vi "Create Message - Trigger Only.vi"(7 "optional settings":T2={"Protection"=enum."None", "Enable Periodic Default"=FALSE, "Trigger Channel refnum"=18446744073709551615} {"Trigger Channel refnum" format="%x"}, 8 "error in (no error)":errorcluster, 10 "message name":string, 11 "message group refnum in":T1=18446744073709551615 format="%.0x") -> (0 "error out":errorcluster, 2 "message refnum out":T1 format="%.0x", 3 "message group refnum out":T1 format="%.0x")   [LabVIEW 2020, in "Instrument Addon Scripting API.lvlib"]
doc: "Creates a new message section that sets the Generation Type as Trigger Only. \n\nTrigger Only is best used for single event messages, such as setting the instrument configuration at the beginning of a test."
uses:
  Instrument Addon Scripting API.lvlib
  TypeDefs/Message Settings.ctl
  TypeDefs/Protection Types.ctl
  <vilib>/NI VeriStand/Custom Device API/Custom Device Item Ref.ctl
  <vilib>/NI VeriStand/Custom Device API/Custom Device Channel.ctl
  <vilib>/NI VeriStand/Custom Device API/Custom Device Channel Type.ctl
  Addon/Addon Shared/Types/Message Generation Type.ctl
  <vilib>/NI VeriStand/Custom Device API/Custom Device API.lvlib
  Addon/Addon Shared/Instrument Addon Shared.lvlib
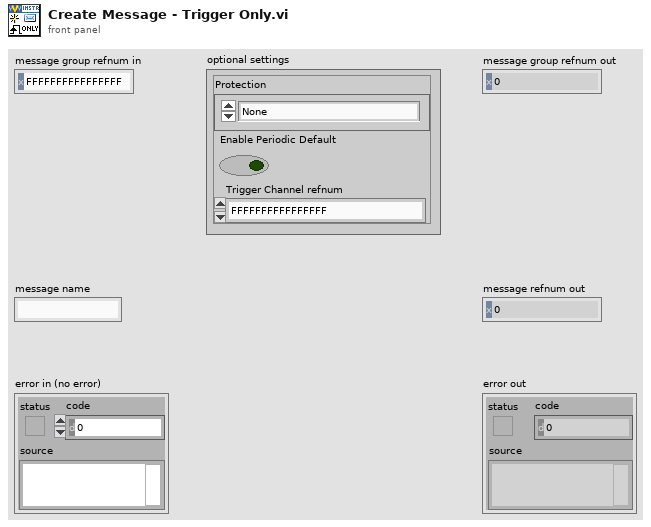
[diagram p1: front panel]
types:
  T1 = typedef "Custom Device API.lvlib/Custom Device Item Ref.ctl" = u64
  T2 = typedef "Instrument Addon Scripting API.lvlib/Message Settings.ctl" = cluster{"Protection":T3, "Enable Periodic Default":bool, "Trigger Channel refnum":u64}
  T3 = typedef "Instrument Addon Scripting API.lvlib/Protection Types.ctl" = enum16{"None", "CRC-32", "Checksum U16", "Checksum U32", "Checksum U8"}
  T4 = typedef "Instrument Addon Shared.lvlib/Message Generation Type.ctl" = enum16{"Trigger Only", "Periodic & Trigger", "Value Change & Trigger"}
  T5 = typedef "Custom Device API.lvlib/Custom Device Channel.ctl" = cluster{"Type":T6, "Units":string, "Default Value":dbl, "Faultable":bool, "Scalable":bool}
  T6 = typedef "Custom Device API.lvlib/Custom Device Channel Type.ctl" = enum16{"Input", "Output"}
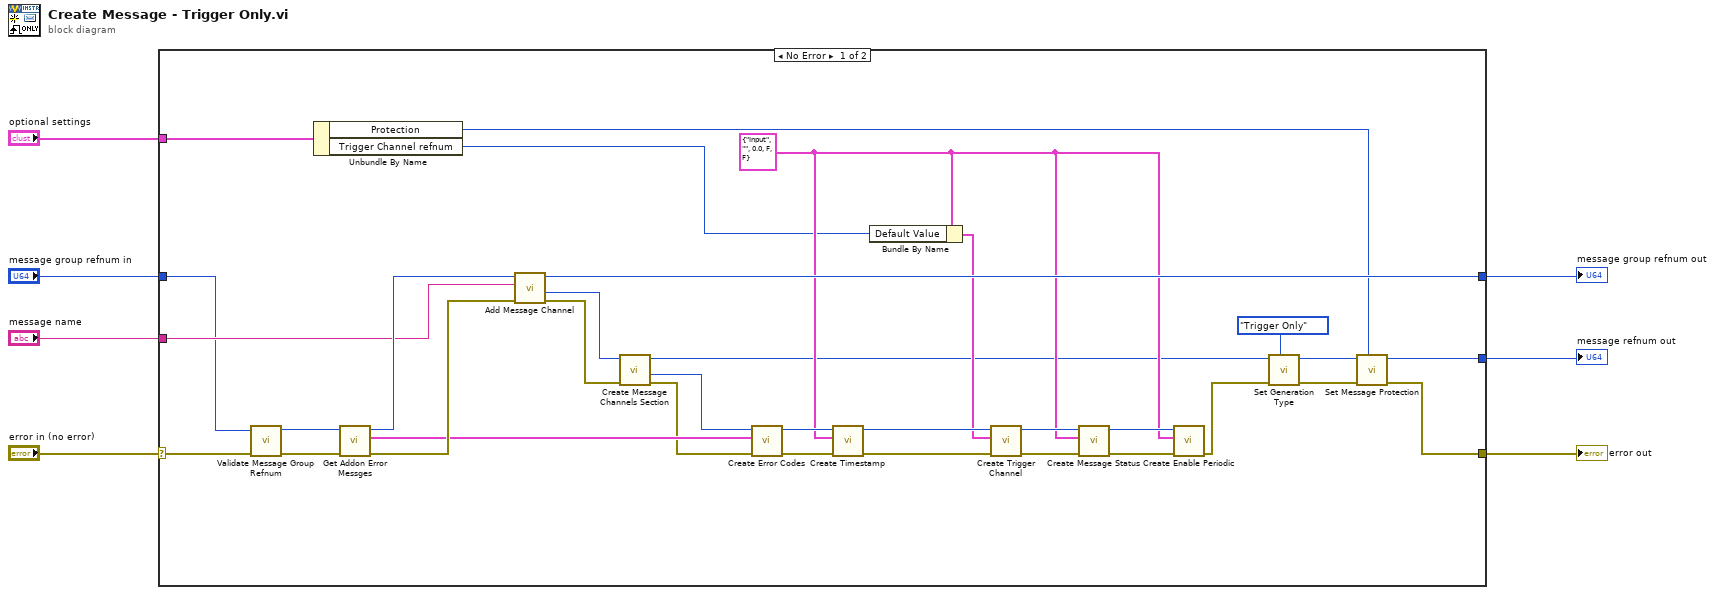
[diagram p0: block diagram]
diagram:
  n1 = case shown="No Error" "error in (no error)" {
    selector: "error in (no error)" -> [w10 w42]
    tunnel: "message group refnum in" -> [w9 w41]
    tunnel: "optional settings" -> [w36 _]
    tunnel: [w32 w41] -> w3
    tunnel: "message name" -> [w29 _]
    tunnel: [w24 _] -> w2
    tunnel: [w23 w42] -> w7
    frame No Error {
      w16 = T5 {"Type"=enum."Input", "Units"="", "Default Value"=0.0, "Faultable"=FALSE, "Scalable"=FALSE} ("Channel")
      n2 = call "Validate Message Group Refnum.vi"("error in (no error)"=w10, "message group refnum in"=w9) -> ("error out"=w11:errorcluster, "message group refnum out"=w8:T1)  [unwired: 8 in]
      n3 = Unbundle By Name(w36) -> ("Protection"=w25:T3, "Trigger Channel refnum"=w14:u64)
      n4 = call "Get Addon Error Messges.vi"("error in (no error)"=w11, "Message Group in"=w8) -> ("error out"=w37:errorcluster, "Error Messages out"=w34:cluster{"Code":i32, "String":string}[], "Message Group out"=w33:u64)  [unwired: 7 in]
      n5 = call "Add Message Channel.vi"("error in (no error)"=w37, "Message Name"=w29, "Message Group in"=w33) -> ("error out"=w40:errorcluster, "Message out"=w35:T1, "Message Group out"=w32:T1)  [unwired: 6 in]
      n6 = call "Create Message Channels Section.vi"("error in (no error)"=w40, "Message in"=w35) -> ("error out"=w31:errorcluster, "Message Channels Section out"=w30:T1, "Message out"=w12:T1)  [unwired: 7 in]
      n7 = call "Create Error Codes.vi"("error in (no error)"=w31, "Error Codes"=w34, "Message Channels Section in"=w30) -> ("error out"=w22:errorcluster, "Message Channels Section out"=w21:T1)  [unwired: 7 in]
      n8 = call "Create Timestamp.vi"("error in (no error)"=w22, "Channel Paramters"=w16, "Message Channels Section in"=w21) -> ("error out"=w20:errorcluster, "Message Channels Section out"=w19:T1)  [unwired: 6 in, 1 out]
      n9 = Bundle By Name(cluster=w16, "Default Value"=w14) -> (w15:T5)
      n10 = call "Create Trigger Channel.vi"("error in (no error)"=w20, "Channel Parameters"=w15, "Message Channels Section in"=w19) -> ("error out"=w18:errorcluster, "Message Channels Section out"=w17:T1)  [unwired: 6 in, 1 out]
      n11 = call "Create Message Status.vi"("error in (no error)"=w18, "Channel Paramters"=w16, "Message Channels Section in"=w17) -> ("error out"=w39:errorcluster, "Message Channels Section out"=w38:T1)  [unwired: 7 in]
      n12 = call "Create Enable Periodic.vi"("error in (no error)"=w39, "Channel Parameters"=w16, "Message Channels Section in"=w38) -> ("error out"=w13:errorcluster)  [unwired: 7 in, 1 out]
      n13 = call "Set Generation Type.vi"("Generation Type"=Message_Generation_Type."Trigger Only", "error in (no error)"=w13, "Message in"=w12) -> ("error out"=w27:errorcluster, "Message out"=w26:T1)  [unwired: 7 in]
      n14 = call "Set Message Protection.vi"("Protection Type"=w25, "error in (no error)"=w27, "Message in"=w26) -> ("error out"=w23:errorcluster, "Message out"=w24:T1)  [unwired: 7 in]
    }
    frame Error {
    }
  }
  "error out" <- w7
  "message group refnum out" <- w3
  "message refnum out" <- w2
